vi "Q_ini.vi"(7 "Parameterek":T1={"rholevego"=0.0, "Vlevego"=0.0, "Mlevego"=0.0, "clevego"=1.0, "rho PCM"=1100.0, "rho kulso"=28.3, "Dkulso"=0.1, "nkulso"=10, "dkulso"=0.0, "vkulso"=0.0, "rho kozepso"=28.3, "Dkozepso"=0.06, "nkozepso"=6, "dkozepso"=0.0, "vkozepso"=0.0, "mkozepso"=0.0, "mkulso"=0.0, "rho belso"=28.3, "Dbelso"=0.1, "nbelso"=10, "dbelso"=0.0, "vbelso"=0.0, "mbelso"=0.0, "Xpcm_kulso"=0.3, "Xpcm_belso"=0.3, "mpcm_kulso"=0.0, "mpcm_belso"=0.0, "mkulso_pcm"=0.0, "mbelso_pcm"=0.0, "ckulso"=1.13, "ckozepso"=1.13, "cbelso"=1.13, "cpcm_szilard"=1.9, "cpcm_foly"=1.5, "ckulso_Topalatt"=0.0, "cbelso_Topalatt"=0.0, "ckulso_Topfelett"=0.0, "cbelso_Topfelett"=0.0, "hpcm_olv"=140.0, "ckulso_eff_Tolv"=0.0, "cbelso_eff_Tolv"=0.0, "Qkulso_op_also"=0.0, "Qkulso_op_felso"=0.0, "Qbelso_op_also"=0.0, "Qbelso_op_felso"=0.0, "lambda_kulso"=5e-05, "lambda_kozepso"=5e-05, "lambda_belso"=5e-05, "lambda_pcm"=0.00018, "VXpcm_kulso"=0.0, "VXpcm_belso"=0.0, "lambda_kulsoPCM"=0.0, "lambda_belsoPCM"=0.0, "Alfa_kulso"=0.015, "Alfa_belso"=0.006, "Alfa_kont"=0.03, "Top_also"=24.0, "Top_felso"=28.0, "cpcm_olvnelkul"=0.0, "Tbelsolevego_0"=22.0}, 8 "T_belso_0":dbl, 9 "T_kozepso_0":dbl, 10 "T_kulso_0":dbl) -> (0 "Q_belso_0_vektor":dbl[](array[numeric]), 1 "Q_kozepso_0_vektor":dbl[](array[numeric]), 2 "Q_kulso_0 vektor":dbl[](array[numeric]))   [LabVIEW 2013]
uses:
  Parameterek.ctl
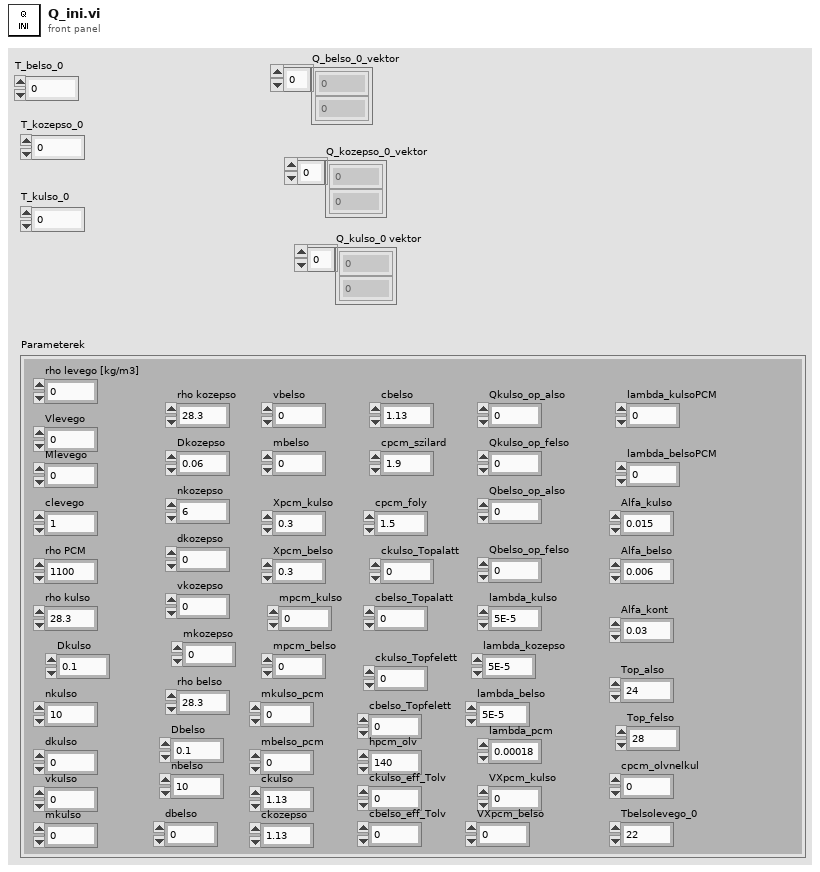
[diagram p1: front panel]
types:
  T1 = typedef "Parameterek.ctl" = cluster{"rholevego":dbl, "Vlevego":dbl, "Mlevego":dbl, "clevego":dbl, "rho PCM":dbl, "rho kulso":dbl, "Dkulso":dbl, "nkulso":i32, "dkulso":dbl, "vkulso":dbl, "rho kozepso":dbl, "Dkozepso":dbl, "nkozepso":i32, "dkozepso":dbl, "vkozepso":dbl, "mkozepso":dbl, "mkulso":dbl, "rho belso":dbl, "Dbelso":dbl, "nbelso":i32, "dbelso":dbl, "vbelso":dbl, "mbelso":dbl, "Xpcm_kulso":dbl, "Xpcm_belso":dbl, "mpcm_kulso":dbl, "mpcm_belso":dbl, "mkulso_pcm":dbl, "mbelso_pcm":dbl, "ckulso":dbl, "ckozepso":dbl, "cbelso":dbl, "cpcm_szilard":dbl, "cpcm_foly":dbl, "ckulso_Topalatt":dbl, "cbelso_Topalatt":dbl, "ckulso_Topfelett":dbl, "cbelso_Topfelett":dbl, "hpcm_olv":dbl, "ckulso_eff_Tolv":dbl, "cbelso_eff_Tolv":dbl, "Qkulso_op_also":dbl, "Qkulso_op_felso":dbl, "Qbelso_op_also":dbl, "Qbelso_op_felso":dbl, "lambda_kulso":dbl, "lambda_kozepso":dbl, "lambda_belso":dbl, "lambda_pcm":dbl, "VXpcm_kulso":dbl, "VXpcm_belso":dbl, "lambda_kulsoPCM":dbl, "lambda_belsoPCM":dbl, "Alfa_kulso":dbl, "Alfa_belso":dbl, "Alfa_kont":dbl, "Top_also":dbl, "Top_felso":dbl, "cpcm_olvnelkul":dbl, "Tbelsolevego_0":dbl}
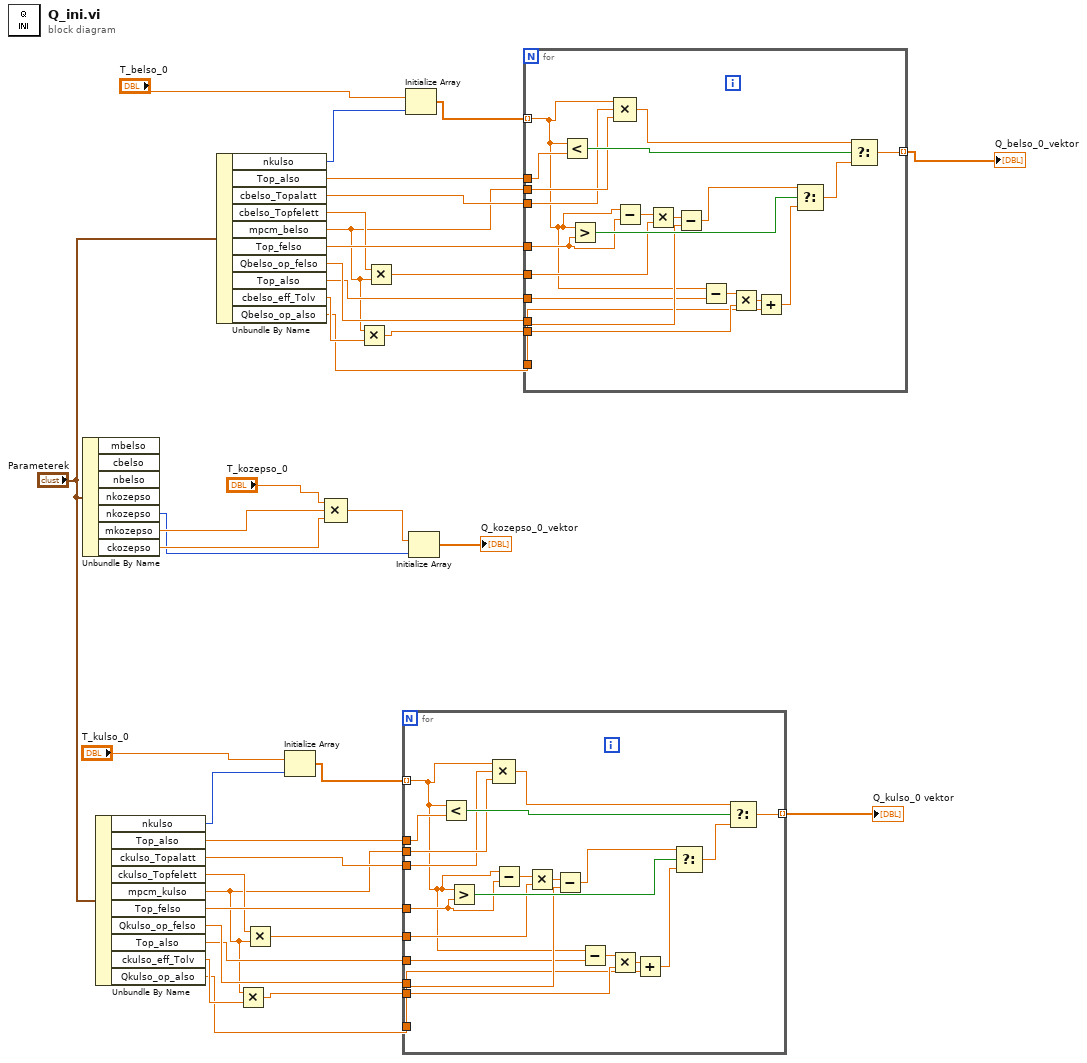
[diagram p0: block diagram]
diagram:
  n1 = Unbundle By Name("Parameterek") -> ("nkozepso"=w22:i32, "mkozepso"=w34:dbl, "ckozepso"=w33:dbl)  [unwired: 4 out]
  n2 = Unbundle By Name("Parameterek") -> ("nkulso"=w23:i32, "Top_also"=w30:dbl, "ckulso_Topalatt"=w29:dbl, "ckulso_Topfelett"=w27:dbl, "mpcm_kulso"=w19:dbl, "Top_felso"=w28:dbl, "Qkulso_op_felso"=w25:dbl, "Top_also"=w21:dbl, "ckulso_eff_Tolv"=w20:dbl, "Qkulso_op_also"=w17:dbl)
  n3 = Unbundle By Name("Parameterek") -> ("nkulso"=w9:i32, "Top_also"=w15:dbl, "cbelso_Topalatt"=w14:dbl, "cbelso_Topfelett"=w12:dbl, "mpcm_belso"=w6:dbl, "Top_felso"=w13:dbl, "Qbelso_op_felso"=w10:dbl, "Top_also"=w8:dbl, "cbelso_eff_Tolv"=w7:dbl, "Qbelso_op_also"=w4:dbl)
  n4 = Multiply(x=w19, y=w20) -> (x*y=w18:dbl)
  n5 = Multiply(x=w27, y=w19) -> (x*y=w26:dbl)
  n6 = Initialize Array("T_kulso_0", w23) -> (w31:dbl[])
  n7 = Compound Arithmetic op=MULTIPLY("T_kozepso_0", w34, w33) -> (w35:dbl)
  n8 = Multiply(x=w6, y=w7) -> (x*y=w5:dbl)
  n9 = Multiply(x=w12, y=w6) -> (x*y=w11:dbl)
  n10 = for {
    tunnel: w31 -> [w44] mode=indexing
    tunnel: w30 -> [w58]
    tunnel: w19 -> [w55]
    tunnel: w29 -> [w54]
    tunnel: w28 -> [w51]
    tunnel: w26 -> [w49]
    tunnel: w25 -> [w47]
    tunnel: [w45] -> w24 mode=indexing
    tunnel: w21 -> [w43]
    tunnel: w18 -> [w41]
    tunnel: w17 -> [w39]
    n11 = Less?(x=w44, y=w58) -> (x < y?=w57:bool)
    n12 = Greater?(x=w44, y=w51) -> (0:w52:bool)
    n13 = Compound Arithmetic op=MULTIPLY(w44, w54, w55) -> (w56:dbl)
    n14 = Subtract(x=w44, y=w51) -> (x-y=w50:dbl)
    n15 = Multiply(x=w50, y=w49) -> (x*y=w48:dbl)
    n16 = Subtract(x=w48, y=w47) -> (x-y=w46:dbl)
    n17 = Subtract(x=w44, y=w43) -> (x-y=w42:dbl)
    n18 = Multiply(x=w42, y=w41) -> (x*y=w40:dbl)
    n19 = Add(x=w40, y=w39) -> (x+y=w38:dbl)
    n20 = Select(t=w46, s=w52, f=w38) -> (s? t:f=w53:dbl)
    n21 = Select(t=w56, s=w57, f=w53) -> (s? t:f=w45:dbl)
  }
  "Q_kulso_0 vektor" <- w24
  n22 = Initialize Array("T_belso_0", w9) -> (w16:dbl[])
  n23 = Initialize Array(w35, w22) -> (→"Q_kozepso_0_vektor":dbl[])
  n24 = for {
    tunnel: w16 -> [w65] mode=indexing
    tunnel: w15 -> [w79]
    tunnel: w6 -> [w76]
    tunnel: w14 -> [w75]
    tunnel: w13 -> [w72]
    tunnel: w11 -> [w70]
    tunnel: w10 -> [w68]
    tunnel: [w66] -> w2 mode=indexing
    tunnel: w8 -> [w64]
    tunnel: w5 -> [w62]
    tunnel: w4 -> [w60]
    n25 = Less?(x=w65, y=w79) -> (x < y?=w78:bool)
    n26 = Greater?(x=w65, y=w72) -> (0:w73:bool)
    n27 = Compound Arithmetic op=MULTIPLY(w65, w75, w76) -> (w77:dbl)
    n28 = Subtract(x=w65, y=w72) -> (x-y=w71:dbl)
    n29 = Multiply(x=w71, y=w70) -> (x*y=w69:dbl)
    n30 = Subtract(x=w69, y=w68) -> (x-y=w67:dbl)
    n31 = Subtract(x=w65, y=w64) -> (x-y=w63:dbl)
    n32 = Multiply(x=w63, y=w62) -> (x*y=w61:dbl)
    n33 = Add(x=w61, y=w60) -> (x+y=w59:dbl)
    n34 = Select(t=w67, s=w73, f=w59) -> (s? t:f=w74:dbl)
    n35 = Select(t=w77, s=w78, f=w74) -> (s? t:f=w66:dbl)
  }
  "Q_belso_0_vektor" <- w2
